vi "subSetAllParameters.vi"(8 "error in (no error)":errorcluster, 9 "Parameters":map{string, string}(c390), 11 "CDependencyInspection in":refnum<class "CDependencyInspection.lvclass">) -> (0 "error out":errorcluster, 2 "Config file path":path, 3 "CDependencyInspection out":refnum<class "CDependencyInspection.lvclass">)   [LabVIEW 2020, in "DependencyInspection.lvlib" / "CDependencyInspection.lvclass"]
uses:
  CDependencyInspection.lvclass
  CDependencyInspection.lvclass/CDependencyInspection.ctl
  CItemMatch/TypeDefs/Field.ctl
  CItemMatch/TypeDefs/ComparisonType.ctl
  cd45eb2e-2d50-4faa-92ce-3e0260f2586f.vi
  0d8f8697-a6f5-4498-9b4d-382727ecc55d.vi
  7677e2e5-d603-4cb1-88ff-37031b5799cc.vi
  36d449e9-9903-44ca-ae78-9787cc487df7.vi
  CItemMatch/CItemMatch.lvclass
  CommonHelpers/CommonHelpers.lvlib
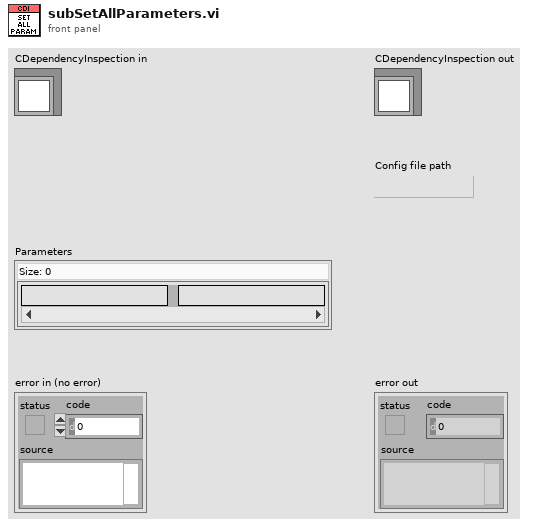
[diagram p1: front panel]
types:
  T1 = typedef "DependencyInspection.lvlib/CItemMatch.lvclass/Field.ctl" = enum16{"Name", "Qualified name", "Path"}
  T2 = typedef "DependencyInspection.lvlib/CItemMatch.lvclass/ComparisonType.ctl" = enum16{"None", "Ends with", "Equals", "Not equal", "Starts with", "Contains", "Matches pattern"}
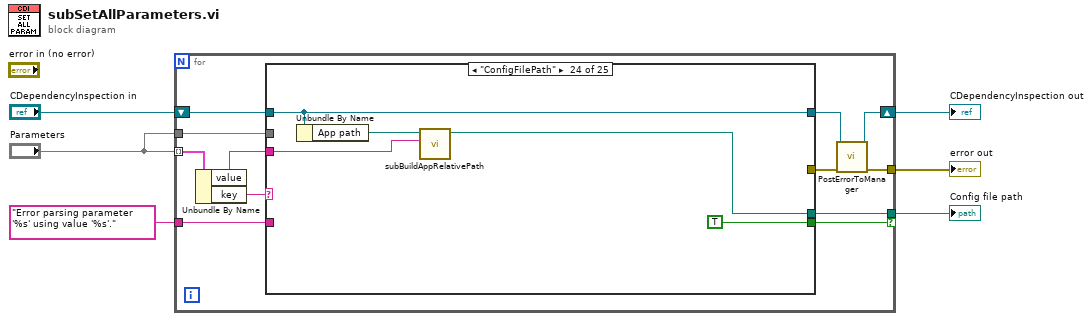
[diagram p0: block diagram]
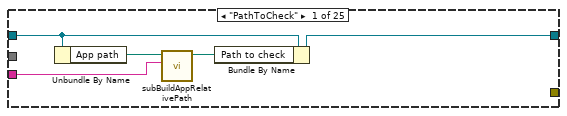
[diagram p2: hidden frame]
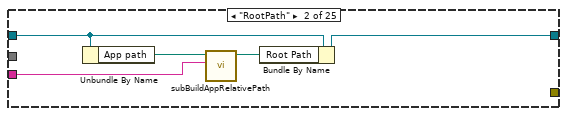
[diagram p3: hidden frame]
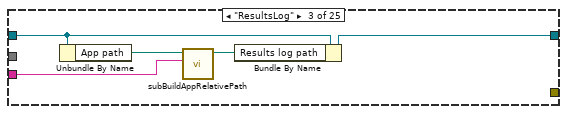
[diagram p4: hidden frame]
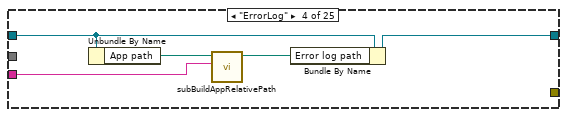
[diagram p5: hidden frame]
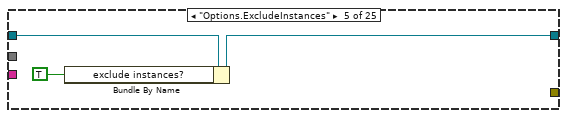
[diagram p6: hidden frame]
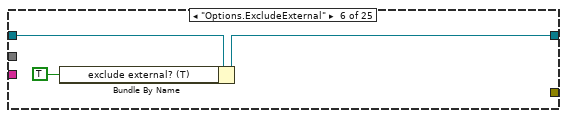
[diagram p7: hidden frame]
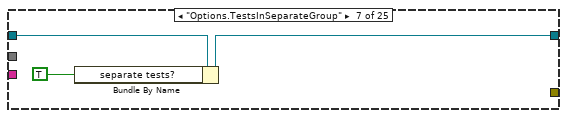
[diagram p8: hidden frame]
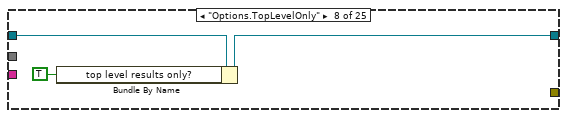
[diagram p9: hidden frame]
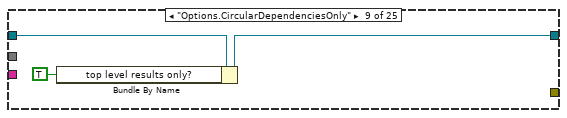
[diagram p10: hidden frame]
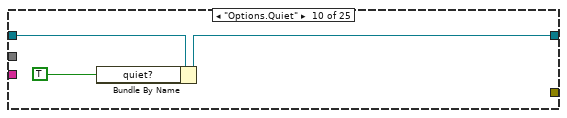
[diagram p11: hidden frame]
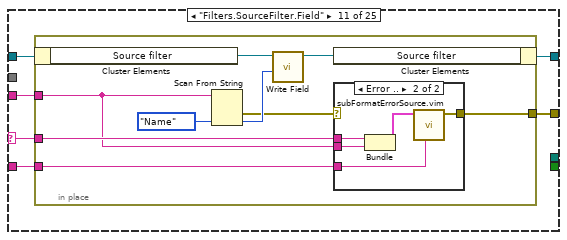
[diagram p12: hidden frame]
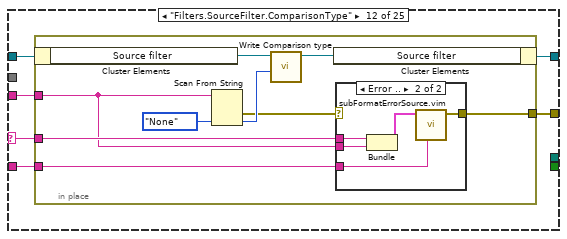
[diagram p14: hidden frame]
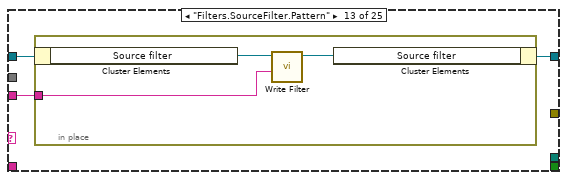
[diagram p16: hidden frame]
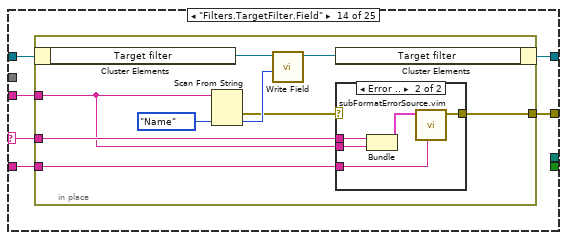
[diagram p17: hidden frame]
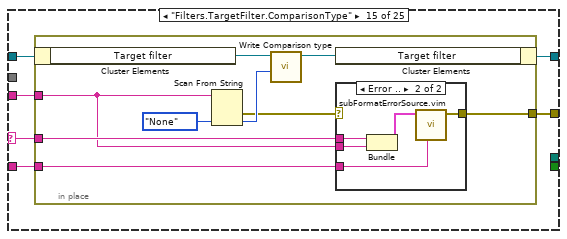
[diagram p19: hidden frame]
diagram:
  n1 = for {
    tunnel: "Parameters" -> [w10] mode=indexing
    tunnel: [w17] -> w5 if=w7
    tunnel: "Error parsing parameter '%s' using value '%s'." ("format string") -> [w16]
    tunnel: [w12] -> w2
    shift-right: [w14] -> w3
    shift-left: "CDependencyInspection in" -> [w18]
    tunnel: "Parameters" -> [w11]
    n2 = Unbundle By Name(w10) -> ("value"=w8:string, "key"=w9:string)
    n3 = case shown="\"ConfigFilePath\"" w9 {
      selector: w9 -> [_ _ _ _ _ _ _ _ _ _ w57 w78 _ w105 w127 _ _ _ _ _ _ _ _ _ _]
      tunnel: w18 -> [w21 w25 w31 w36 w41 w44 w47 w50 w53 w56 w62 w83 w101 w110 w131 w149 w155 w158 w161 w164 w169 w172 w175 w180 w183]
      tunnel: w8 -> [w19 w26 w30 w34 _ _ _ _ _ _ w60 w81 w99 w108 w129 w147 _ w156 w159 w162 w167 w170 w173 w182 _]
      tunnel: [w23 w28 w33 w38 w40 w43 w46 w49 w52 w55 w61 w82 w100 w109 w130 w148 w154 w157 w160 w166 w168 w171 w177 w180 w183] -> w15
      tunnel: [_ _ _ _ _ _ _ _ _ _ w59 w80 _ w107 w128 _ _ _ _ _ _ _ _ _ _] -> w13
      tunnel: [_ _ _ _ _ _ _ _ _ _ _ _ _ _ _ _ _ _ _ _ _ _ _ w181 _] -> w17
      tunnel: w16 -> [_ _ _ _ _ _ _ _ _ _ w58 w79 _ w106 w126 _ _ _ _ _ _ _ _ _ _]
      tunnel: w11 -> [_ _ _ _ _ _ _ _ _ _ _ _ _ _ _ _ _ _ _ _ _ _ _ _ _]
      tunnel: [_ _ _ _ _ _ _ _ _ _ _ _ _ _ _ _ _ _ _ _ _ _ _ TRUE _] -> w7
      frame "PathToCheck" {
        n4 = Unbundle By Name(w21) -> ("App path"=w22:path)
        n5 = call "subBuildAppRelativePath.vi"("String path"=w19, "App path"=w22) -> ("appended path"=w20:path)  [unwired: 9 in]
        n6 = Bundle By Name(cluster=w21, "Path to check"=w20) -> (w23:refnum<class "CDependencyInspection.lvclass">)
      }
      frame "RootPath" {
        n7 = Unbundle By Name(w25) -> ("App path"=w27:path)
        n8 = call "subBuildAppRelativePath.vi"("String path"=w26, "App path"=w27) -> ("appended path"=w24:path)  [unwired: 9 in]
        n9 = Bundle By Name(cluster=w25, "Root Path"=w24) -> (w28:refnum<class "CDependencyInspection.lvclass">)
      }
      frame "ResultsLog" {
        n10 = Unbundle By Name(w31) -> ("App path"=w32:path)
        n11 = call "subBuildAppRelativePath.vi"("String path"=w30, "App path"=w32) -> ("appended path"=w29:path)  [unwired: 9 in]
        n12 = Bundle By Name(cluster=w31, "Results log path"=w29) -> (w33:refnum<class "CDependencyInspection.lvclass">)
      }
      frame "ErrorLog" {
        n13 = Unbundle By Name(w36) -> ("App path"=w37:path)
        n14 = call "subBuildAppRelativePath.vi"("String path"=w34, "App path"=w37) -> ("appended path"=w35:path)  [unwired: 9 in]
        n15 = Bundle By Name(cluster=w36, "Error log path"=w35) -> (w38:refnum<class "CDependencyInspection.lvclass">)
      }
      frame "Options.ExcludeInstances" {
        n16 = Bundle By Name(cluster=w41, "exclude instances?"=TRUE ("Options.exclude instances?")) -> (w40:refnum<class "CDependencyInspection.lvclass">)
      }
      frame "Options.ExcludeExternal" {
        n17 = Bundle By Name(cluster=w44, "exclude external? (T)"=TRUE ("Options.exclude instances?")) -> (w43:refnum<class "CDependencyInspection.lvclass">)
      }
      frame "Options.TestsInSeparateGroup" {
        n18 = Bundle By Name(cluster=w47, "separate tests?"=TRUE ("Options.exclude instances?")) -> (w46:refnum<class "CDependencyInspection.lvclass">)
      }
      frame "Options.TopLevelOnly" {
        n19 = Bundle By Name(cluster=w50, "top level results only?"=TRUE ("Options.exclude instances?")) -> (w49:refnum<class "CDependencyInspection.lvclass">)
      }
      frame "Options.CircularDependenciesOnly" {
        n20 = Bundle By Name(cluster=w53, "top level results only?"=TRUE ("Options.exclude instances?")) -> (w52:refnum<class "CDependencyInspection.lvclass">)
      }
      frame "Options.Quiet" {
        n21 = Bundle By Name(cluster=w56, "quiet?"=TRUE ("Options.exclude instances?")) -> (w55:refnum<class "CDependencyInspection.lvclass">)
      }
      frame "Filters.SourceFilter.Field" {
        n22 = in-place {
          in-place-border: w60 -> [w63]
          in-place-border: [w66] -> w59
          in-place-border: w58 -> [w65]
          in-place-border: w57 -> [w64]
          n23 = in-place-cluster #1(w62) -> ("Source filter"=w71:refnum<class "CItemMatch.lvclass">)
          n24 = Scan From String(input string=w63, default 1=Field."Name" ("Field")) -> (error out=w67:errorcluster, output 1=w68:T1)  [unwired: 3 in, 2 out]
          n25 = call-dynamic "Write Field.vi"("Field"=w68, "CItemMatch in"=w71) -> ("CItemMatch out"=w70:refnum<class "CItemMatch.lvclass">)  [unwired: 9 in]
          n26 = in-place-cluster #1("Source filter"=w70) -> (w61:refnum<class "CDependencyInspection.lvclass">)
          n27 = case shown="Error .." w67 {
            selector: w67 -> [w72 _]
            tunnel: [w72 w77] -> w66
            tunnel: w65 -> [_ w76]
            tunnel: w64 -> [_ w75]
            tunnel: w63 -> [_ w74]
            frame No Error {
            }
            frame Error {
              n28 = Bundle(w75, "value"=w74) -> (w73:cluster{string, "value":string})  [unwired: 1 in]
              n29 = call "subFormatErrorSource.vim"("format string"=w76, "Parameter cluster"=w73) -> ("Error out"=w77:errorcluster)  [unwired: 9 in]
            }
          }
        }
      }
      frame "Filters.SourceFilter.ComparisonType" {
        n30 = in-place {
          in-place-border: w81 -> [w85]
          in-place-border: [w84] -> w80
          in-place-border: w79 -> [w87]
          in-place-border: w78 -> [w86]
          n31 = in-place-cluster #2(w83) -> ("Source filter"=w92:refnum<class "CItemMatch.lvclass">)
          n32 = Scan From String(input string=w85, default 1=ComparisonType."None" ("Comparison type")) -> (error out=w88:errorcluster, output 1=w89:T2)  [unwired: 3 in, 2 out]
          n33 = call-dynamic "Write Comparison type.vi"("Comparison type"=w89, "CItemMatch in"=w92) -> ("CItemMatch out"=w91:refnum<class "CItemMatch.lvclass">)  [unwired: 9 in]
          n34 = in-place-cluster #2("Source filter"=w91) -> (w82:refnum<class "CDependencyInspection.lvclass">)
          n35 = case shown="Error .." w88 {
            selector: w88 -> [w93 _]
            tunnel: [w93 w98] -> w84
            tunnel: w87 -> [_ w97]
            tunnel: w86 -> [_ w96]
            tunnel: w85 -> [_ w95]
            frame No Error {
            }
            frame Error {
              n36 = Bundle(w96, "value"=w95) -> (w94:cluster{string, "value":string})  [unwired: 1 in]
              n37 = call "subFormatErrorSource.vim"("format string"=w97, "Parameter cluster"=w94) -> ("Error out"=w98:errorcluster)  [unwired: 9 in]
            }
          }
        }
      }
      frame "Filters.SourceFilter.Pattern" {
        n38 = in-place {
          in-place-border: w99 -> [w102]
          n39 = in-place-cluster #3(w101) -> ("Source filter"=w104:refnum<class "CItemMatch.lvclass">)
          n40 = call-dynamic "Write Filter.vi"("Filter"=w102, "CItemMatch in"=w104) -> ("CItemMatch out"=w103:refnum<class "CItemMatch.lvclass">)  [unwired: 9 in]
          n41 = in-place-cluster #3("Source filter"=w103) -> (w100:refnum<class "CDependencyInspection.lvclass">)
        }
      }
      frame "Filters.TargetFilter.Field" {
        n42 = in-place {
          in-place-border: w108 -> [w112]
          in-place-border: [w111] -> w107
          in-place-border: w106 -> [w114]
          in-place-border: w105 -> [w113]
          n43 = in-place-cluster #4(w110) -> ("Target filter"=w119:refnum<class "CItemMatch.lvclass">)
          n44 = Scan From String(input string=w112, default 1=Field."Name" ("Field")) -> (error out=w115:errorcluster, output 1=w116:T1)  [unwired: 3 in, 2 out]
          n45 = call-dynamic "Write Field.vi"("Field"=w116, "CItemMatch in"=w119) -> ("CItemMatch out"=w118:refnum<class "CItemMatch.lvclass">)  [unwired: 9 in]
          n46 = in-place-cluster #4("Target filter"=w118) -> (w109:refnum<class "CDependencyInspection.lvclass">)
          n47 = case shown="Error .." w115 {
            selector: w115 -> [w120 _]
            tunnel: [w120 w125] -> w111
            tunnel: w114 -> [_ w124]
            tunnel: w113 -> [_ w123]
            tunnel: w112 -> [_ w122]
            frame No Error {
            }
            frame Error {
              n48 = Bundle(w123, "value"=w122) -> (w121:cluster{string, "value":string})  [unwired: 1 in]
              n49 = call "subFormatErrorSource.vim"("format string"=w124, "Parameter cluster"=w121) -> ("Error out"=w125:errorcluster)  [unwired: 9 in]
            }
          }
        }
      }
      frame "Filters.TargetFilter.ComparisonType" {
        n50 = in-place {
          in-place-border: w129 -> [w132]
          in-place-border: [w135] -> w128
          in-place-border: w127 -> [w134]
          in-place-border: w126 -> [w133]
          n51 = in-place-cluster #5(w131) -> ("Target filter"=w140:refnum<class "CItemMatch.lvclass">)
          n52 = Scan From String(input string=w132, default 1=ComparisonType."None" ("Comparison type")) -> (error out=w136:errorcluster, output 1=w137:T2)  [unwired: 3 in, 2 out]
          n53 = call-dynamic "Write Comparison type.vi"("Comparison type"=w137, "CItemMatch in"=w140) -> ("CItemMatch out"=w139:refnum<class "CItemMatch.lvclass">)  [unwired: 9 in]
          n54 = in-place-cluster #5("Target filter"=w139) -> (w130:refnum<class "CDependencyInspection.lvclass">)
          n55 = case shown="Error .." w136 {
            selector: w136 -> [w141 _]
            tunnel: [w141 w146] -> w135
            tunnel: w133 -> [_ w145]
            tunnel: w134 -> [_ w144]
            tunnel: w132 -> [_ w143]
            frame No Error {
            }
            frame Error {
              n56 = Bundle(w144, "value"=w143) -> (w142:cluster{string, "value":string})  [unwired: 1 in]
              n57 = call "subFormatErrorSource.vim"("format string"=w145, "Parameter cluster"=w142) -> ("Error out"=w146:errorcluster)  [unwired: 9 in]
            }
          }
        }
      }
      frame "Filters.TargetFilter.Pattern" {
        n58 = in-place {
          in-place-border: w147 -> [w150]
          n59 = in-place-cluster #6(w149) -> ("Target filter"=w152:refnum<class "CItemMatch.lvclass">)
          n60 = call-dynamic "Write Filter.vi"("Filter"=w150, "CItemMatch in"=w152) -> ("CItemMatch out"=w151:refnum<class "CItemMatch.lvclass">)  [unwired: 9 in]
          n61 = in-place-cluster #6("Target filter"=w151) -> (w148:refnum<class "CDependencyInspection.lvclass">)
        }
      }
      frame "Filters.AndConditions" {
        n62 = Bundle By Name(cluster=w155, "AND Condition?"=TRUE ("Options.exclude instances?")) -> (w154:refnum<class "CDependencyInspection.lvclass">)
      }
      frame "RulesParser.Name" {
        n63 = Bundle By Name(cluster=w158, "Name"=w156) -> (w157:refnum<class "CDependencyInspection.lvclass">)
      }
      frame "RulesParser.Parameters" {
        n64 = Bundle By Name(cluster=w161, "Parameters"=w159) -> (w160:refnum<class "CDependencyInspection.lvclass">)
      }
      frame "RulesParser.Path" {
        n65 = Unbundle By Name(w164) -> ("App path"=w165:path)
        n66 = call "subBuildAppRelativePath.vi"("String path"=w162, "App path"=w165) -> ("appended path"=w163:path)  [unwired: 9 in]
        n67 = Bundle By Name(cluster=w164, "Path"=w163) -> (w166:refnum<class "CDependencyInspection.lvclass">)
      }
      frame "Exporter.Name" {
        n68 = Bundle By Name(cluster=w169, "Name"=w167) -> (w168:refnum<class "CDependencyInspection.lvclass">)
      }
      frame "Exporter.Parameters" {
        n69 = Bundle By Name(cluster=w172, "Parameters"=w170) -> (w171:refnum<class "CDependencyInspection.lvclass">)
      }
      frame "Exporter.Path" {
        n70 = Unbundle By Name(w175) -> ("App path"=w176:path)
        n71 = call "subBuildAppRelativePath.vi"("String path"=w173, "App path"=w176) -> ("appended path"=w174:path)  [unwired: 9 in]
        n72 = Bundle By Name(cluster=w175, "Path"=w174) -> (w177:refnum<class "CDependencyInspection.lvclass">)
      }
      frame "ConfigFilePath" {
        n73 = Unbundle By Name(w180) -> ("App path"=w179:path)
        n74 = call "subBuildAppRelativePath.vi"("String path"=w182, "App path"=w179) -> ("appended path"=w181:path)  [unwired: 9 in]
      }
      frame Default {
        # "error"
      }
    }
    n75 = call-dynamic "PostErrorToManager.vi"("error in (no error)"=w13, "CDependencyInspection in"=w15) -> ("error out"=w12:errorcluster, "CDependencyInspection out"=w14:refnum<class "CDependencyInspection.lvclass">)  [unwired: 8 in]
  }
  "error out" <- w2
  "CDependencyInspection out" <- w3
  "Config file path" <- w5
